vi "111_Auto.vi"() -> ()   [LabVIEW 2020]
uses:
  Global_Variable/Global.vi
  Global_Variable/A131258.vi
panel:
  out "合格":bool=TRUE
  out "Tab Control":enum32{"力特性", "内泄露", "压销位移力曲线"}(tab)
  out "力特性":cluster{dbl[], dbl[]}[](graph)
  out "内泄露":cluster{dbl[], dbl[]}[](graph)
  out "压力位移曲线":cluster{dbl[], dbl[]}[](graph)
  in  "判定结果":bool[][](array[boolean])=[[TRUE]]
  in  "STEP":string
  # "力特性试验"
  # "内泄露试验"
  # "压销位移力曲线"
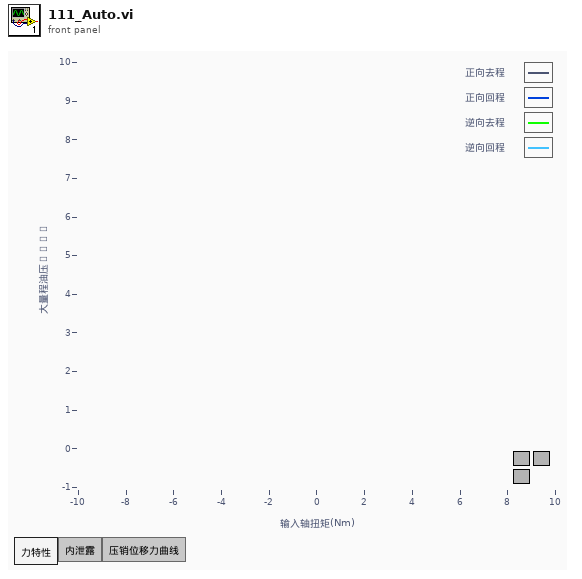
[diagram p1: front panel]
types:
  T1 = typedef "lveventtype.ctl" = enum32{"Null", "Timeout", "Annotation Menu Selection", "Annotation Menu Selection?", "App Instance Close", "App Instance Close?", "Autoscale Range Change", "Bookmark Info Change", "Cell Edit", "Cell Edit?", "Cursor Grab", "Cursor Grab?", "Cursor Menu Selection", "Cursor Menu Selection?", "Cursor Move", "Cursor Release", "Data Change", "Direction Change", "Display State Change", "Drag Ended", "Drag Enter", "Drag Leave", "Drag Over", "Drag Source Update", "Drag Starting", "Drag Starting?", "Drop", "Exec State Change", "Key Down", "Key Down?", "Key Repeat", "Key Repeat?", "Key Up", "Listbox Double Click", "Menu Activation?", "Menu Selection (App)", "Menu Selection? (App)", "Menu Selection (User)", "Mouse Down", "Mouse Down?", "Mouse Enter", "Mouse Leave", "Mouse Move", "Mouse Up", "Mouse Wheel", "NI Security User Change (App)", "Pane Size", "Panel Close", "Panel Close?", "Panel Resize", "Plot Attribute Change", "Scale Range Change", "Shortcut Menu Activation?", "Shortcut Menu Selection (App)", "Shortcut Menu Selection? (App)", "Shortcut Menu Selection (User)", "Tree Double Click", "Tree Drag", "Tree Drag?", "Tree Drop", "Tree Drop?", "Tree Item Close", "Tree Item Close?", "Tree Item Open", "Tree Item Open?", "User Event", "Value Change"}
  T2 = typedef "LVPoint32TypeDef.ctl" = cluster{"Horizontal":i32, "Vertical":i32}
  T3 = cluster{"           对称性":cluster{"下限":dbl, "上限":dbl}, "  正向最大油压":cluster{"下限":dbl, "上限":dbl}, "  逆向最大油压":cluster{"下限":dbl, "上限":dbl}, "定点A正向扭矩":cluster{"下限":dbl, "上限":dbl}, "定点A逆向扭矩":cluster{"下限":dbl, "上限":dbl}, "定点B正向扭矩":cluster{"下限":dbl, "上限":dbl}, "定点B逆向扭矩":cluster{"下限":dbl, "上限":dbl}}
  T4 = cluster{"         对称性":cluster{"下限":dbl, "上限":dbl}, "正向最大角度":cluster{"下限":dbl, "上限":dbl}, "逆向最大角度":cluster{"下限":dbl, "上限":dbl}}
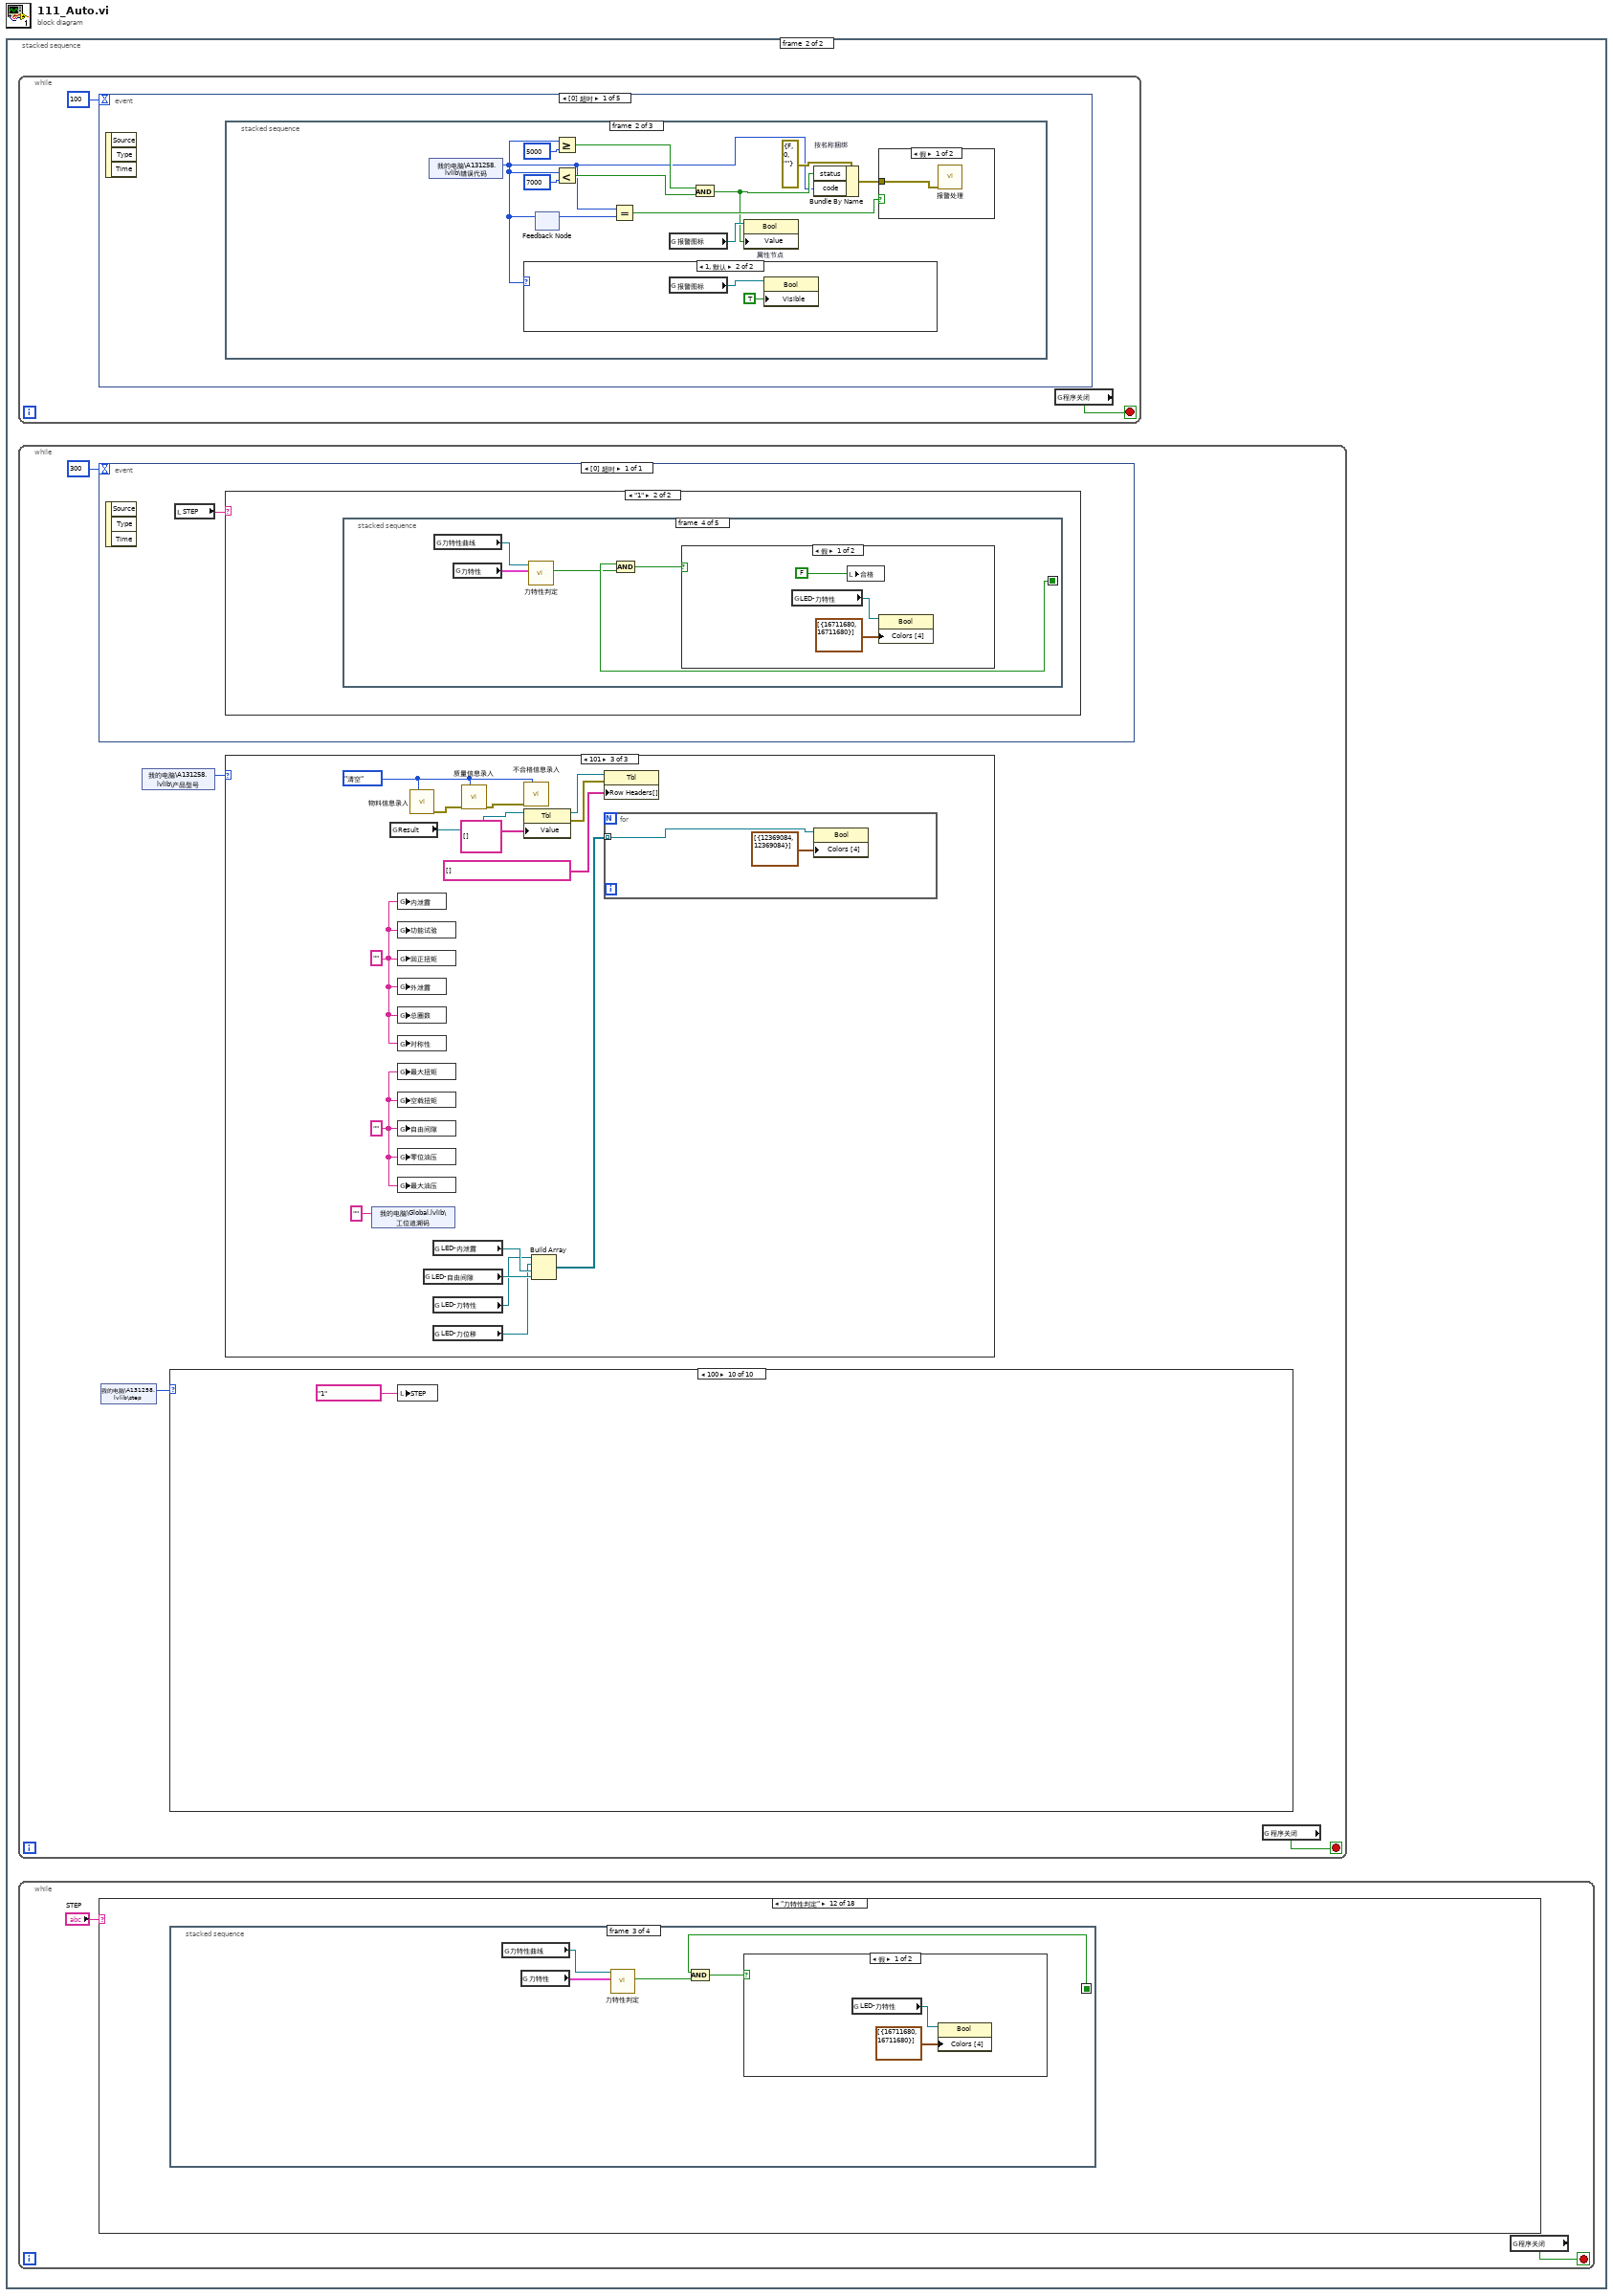
[diagram p0: block diagram]
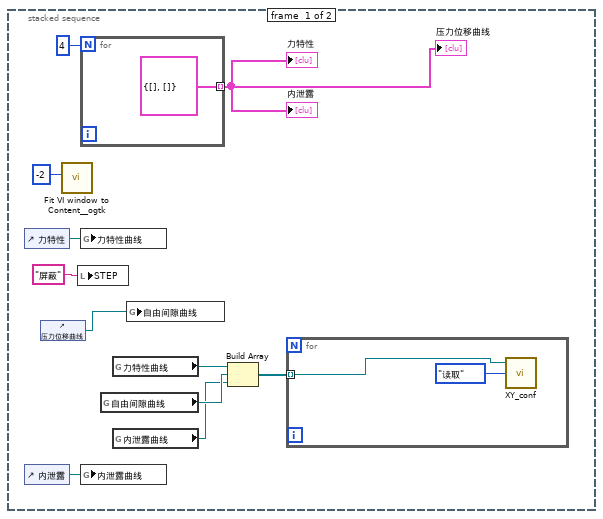
[diagram p2: hidden frame]
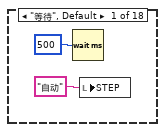
[diagram p3: hidden frame]
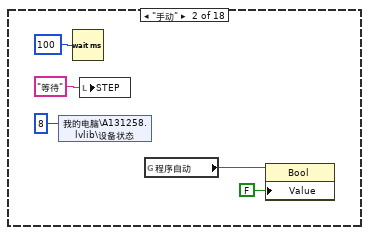
[diagram p4: hidden frame]
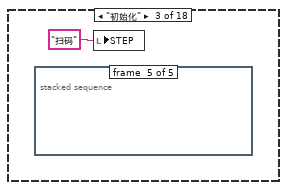
[diagram p5: hidden frame]
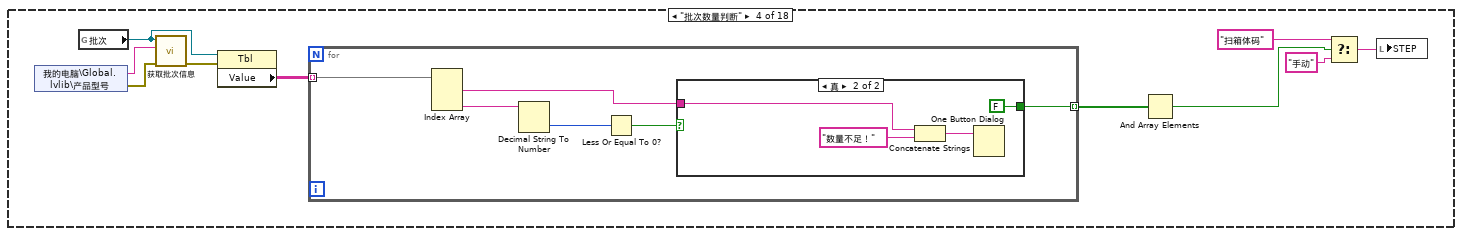
[diagram p10: hidden frame]
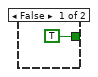
[diagram p11: hidden frame]
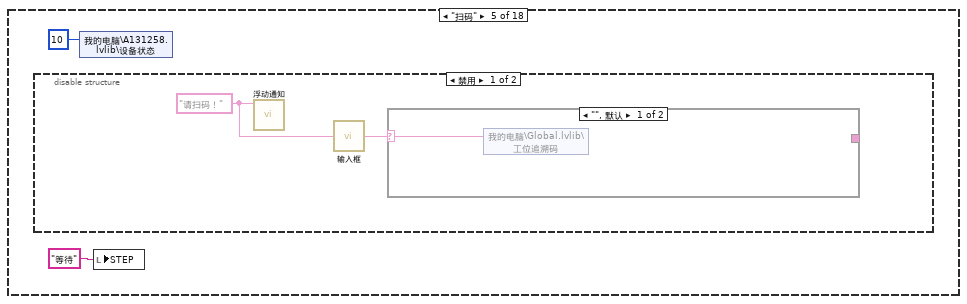
[diagram p12: hidden frame]
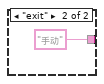
[diagram p13: hidden frame]
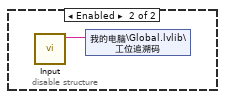
[diagram p14: hidden frame]
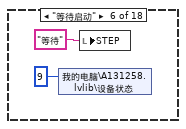
[diagram p15: hidden frame]
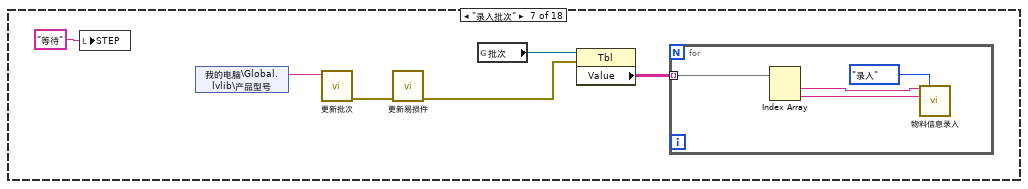
[diagram p16: hidden frame]
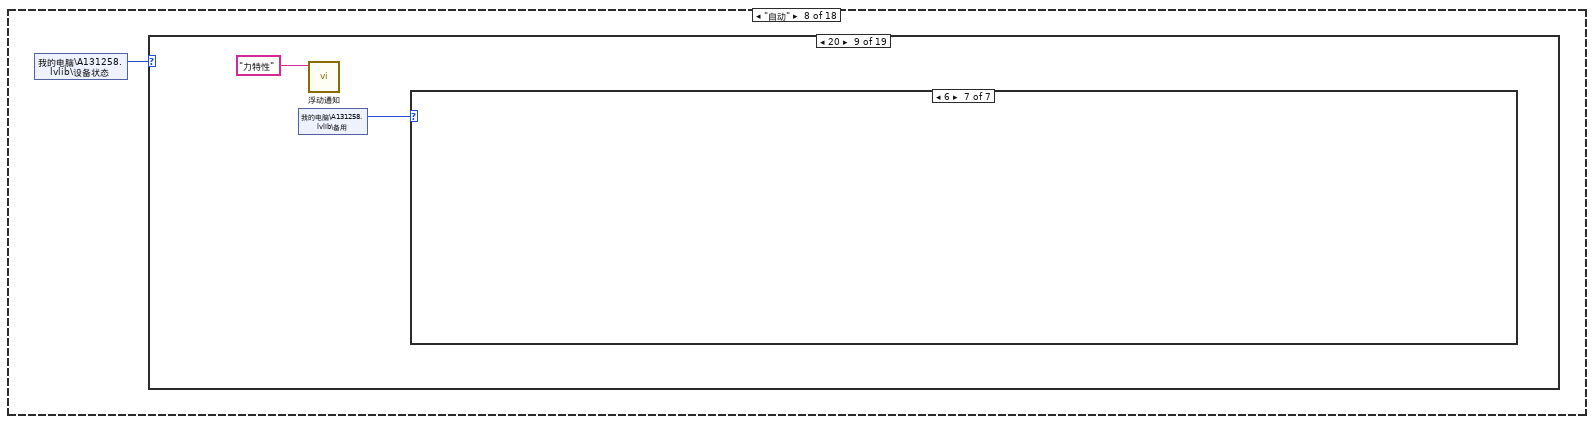
[diagram p17: hidden frame]
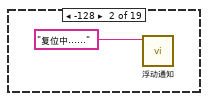
[diagram p19: hidden frame]
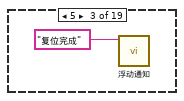
[diagram p20: hidden frame]
diagram:
  n1 = stacked-sequence {
    frame #0 {
      n2 = control-ref of="力特性"() -> (w10:refnum<vi>)
      n3 = control-ref of="内泄露"() -> (w6:refnum<vi>)
      n4 = control-ref of="压力位移曲线"() -> (w9:refnum<vi>)
      n5 = call <userlib>:"Fit VI window to Content__ogtk.vi"("border spacing (2 px)"=-2) -> ()  [unwired: 5 in, 2 out]
      n6 = local write "STEP"("屏蔽" ("STEP")) -> ()
      n7 = for {
        N: 4 -> [_]
        tunnel: [cluster{dbl[], dbl[]} {[], []}] -> w2 mode=indexing
      }
      "压力位移曲线" <- w2
      "力特性" <- w2
      "内泄露" <- w2
      n8 = global write "A131258.vi" "力特性曲线"(w10) -> ()
      n9 = global write "A131258.vi" "内泄露曲线"(w6) -> ()
      n10 = global read "A131258.vi" "自由间隙曲线"() -> (w5:refnum<vi>)
      n11 = global read "A131258.vi" "力特性曲线"() -> (w8:refnum<vi>)
      n12 = global read "A131258.vi" "内泄露曲线"() -> (w4:refnum<vi>)
      n13 = global write "A131258.vi" "自由间隙曲线"(w9) -> ()
      n14 = Build Array(w8, w5, w4) -> (w7:refnum<vi>[])
      n15 = for {
        tunnel: w7 -> [w13] mode=indexing
        n16 = call "XY_conf.vi"("方式"=enum16{"写入", "读取"}."读取", "XY图引用"=w13) -> ()  [unwired: 3 in, 1 out]
      }
    }
    frame #1 {
      n17 = while {
        stop <- w307 stop-if-true
        n18 = event shown="[0] 超时" {
          selector: _ -> [_ _ _ _ _]
          dyn-events: _ -> [_ _ _ _ _]
          timeout: 100 -> [_ _ _ _ _]
          event Timeout {
            n19 = event-data() -> ()  [unwired: 1 in, 3 out]
            n20 = stacked-sequence {
              frame #0 {
                n21 = global read "A131258.vi" "试验项"() -> (→"Tab Control":enum32{"力特性", "内泄露", "压销位移力曲线"})
              }
              frame #1 {
                n22 = shared-variable "我的电脑\\A131258.lvlib\\错误代码"() -> (w310:i16)  [unwired: 1 in, 1 out]
                n23 = case shown="1, 默认" w310 {
                  frame 0 {
                    n24 = global read "Global.vi" "报警图标"() -> (w321:refnum<vi>)
                    n25 = property class="Bool"(reference=w321, "Visible"=FALSE ("可见")) -> ()  [unwired: 1 in, 2 out]
                  }
                  frame 1, Default {
                    n26 = global read "Global.vi" "报警图标"() -> (w324:refnum<vi>)
                    n27 = property class="Bool"(reference=w324, "Visible"=TRUE ("可见")) -> ()  [unwired: 1 in, 2 out]
                  }
                }
                n28 = feedback #1() -> (w320:i16)  [unwired: 1 in]
                n29 = feedback-in #1(w310) -> ()
                n30 = Greater Or Equal?(x=w310, y=i16 5000) -> (x >= y?=w318:bool)
                n31 = Less?(x=w310, y=i16 7000) -> (x < y?=w319:bool)
                n32 = Equal?(x=w310, y=w320) -> (x = y?=w317:bool)
                n33 = global read "Global.vi" "报警图标"() -> (w312:refnum<vi>)
                n34 = And(x=w318, y=w319) -> (x .and. y?=w311:bool)
                n35 = property on="属性节点" class="Bool"(reference=w312, "Value"=w311) -> ()  [unwired: 1 in, 2 out]
                n36 = Bundle By Name "按名称捆绑"(cluster=errorcluster {"status"=FALSE, "code"=0, "source"=""} ("错误常量"), "status"=w311, "code"=w310) -> (w316:errorcluster)
                n37 = case shown="假" w317 {
                  tunnel: w316 -> [w325 _]
                  frame False {
                    n38 = call "报警处理.vi"("错误常量"=w325) -> ()  [unwired: 9 in, 2 out]
                  }
                  frame True {
                  }
                }
              }
              frame #2 {
                n39 = shared-variable "我的电脑\\A131258.lvlib\\自动手动切换"() -> (w326:u16)  [unwired: 1 in, 1 out]
                n40 = case shown="1" w326 {
                  frame 0, Default {
                  }
                  frame 1 {
                    n41 = shared-variable "我的电脑\\A131258.lvlib\\设备状态"() -> (w327:i16)  [unwired: 1 in, 1 out]
                    n42 = case shown="5" w327 {
                      frame Default {
                      }
                      frame 5 {
                      }
                    }
                  }
                }
              }
            }
          }
          event "压力位移曲线", "力特性": Scale Range Change {
            n43 = event-data() -> ("CtlRef"=w328:refnum<vi>)  [unwired: 1 in]
            n44 = call "XY_conf.vi"("方式"=enum16{"写入", "读取"}."写入", "XY图引用"=w328) -> ()  [unwired: 3 in, 1 out]
          }
          event Panel Close {
            n45 = event-data() -> ()  [unwired: 1 in, 4 out]
            n46 = global write "Global.vi" "程序关闭"(TRUE ("程序关闭")) -> ()
          }
          event "压力位移曲线", "力特性": Mouse Enter; "压力位移曲线", "力特性": Mouse Leave; "压力位移曲线", "力特性": Cursor Move {
            n47 = event-data() -> ("CtlRef"=w333:refnum<vi>, "Type"=w331:T1)  [unwired: 1 in]
            n48 = call "CursorShow.vi"("nameShow"=TRUE, "Type"=w331, "Graph"=w333) -> ()  [unwired: 7 in, 2 out]
          }
          event "压力位移曲线", "力特性": Mouse Down {
            n49 = event-data() -> ("CtlRef"=w334:refnum<vi>, "Type"=w337:T1, "Coords"=w336:T2)  [unwired: 1 in]
            n50 = invoke class="XYGraph (严格)" method="Map Coords To XY"(reference=w334, "Coords"=w336) -> ("XY"=w335:cluster{"X":dbl, "Y":dbl})  [unwired: 5 in, 6 out]
            n51 = call "CursorShow.vi"("游标.游标位置"=w335, "Type"=w337, "Graph"=w334) -> ()  [unwired: 7 in, 2 out]
          }
        }
        n52 = global read "Global.vi" "程序关闭"() -> (w307:bool)
      }
      n53 = while {
        stop <- w341 stop-if-true
        n54 = event shown="[0] 超时" {
          selector: _ -> [_]
          dyn-events: _ -> [_]
          timeout: 300 -> [_]
          event Timeout {
            n55 = event-data() -> ()  [unwired: 1 in, 3 out]
            n56 = local read "STEP"() -> (w342:string)
            n57 = case shown="\"1\"" w342 {
              frame "假", Default {
              }
              frame "1" {
                n58 = stacked-sequence {
                  seq-local: [_ _ w358 _ _] -> [_ _ _ w367 _]
                  frame #0 {
                    n59 = local write "STEP"("0" ("STEP")) -> ()
                    n60 = shared-variable "我的电脑\\A131258.lvlib\\step"(i16 101 ("step")) -> ()  [unwired: 1 in, 1 out]
                  }
                  frame #1 {
                    n61 = global read "Global.vi" "Result"() -> (w347:refnum<vi>)
                    n62 = property class="Tbl"(reference=w347) -> (reference out=w350:refnum<vi>, error out=w355:errorcluster, "Row Headers[]"=w348:string[])  [unwired: 1 in]
                    n63 = Build Array (concatenate)(w348, string[] ["力特性"] ("数组")) -> (w349:string[])
                    n64 = property class="Tbl"(reference=w350, error in=w355, "Row Headers[]"=w349) -> (reference out=w351:refnum<vi>, error out=w356:errorcluster)
                    n65 = property class="Tbl"(reference=w351, error in=w356) -> (reference out=w352:refnum<vi>, error out=w357:errorcluster, "Value"=w353:string[][])
                    n66 = Build Array (concatenate)(w353, string[][] [[" "]] ("数组")) -> (w354:string[][])
                    n67 = property class="Tbl"(reference=w352, error in=w357, "Value"=w354) -> ()  [unwired: 2 out]
                  }
                  frame #2 {
                    n68 = shared-variable "我的电脑\\A131258.lvlib\\产品参数"() -> (w362:sgl[])  [unwired: 1 in, 1 out]
                    n69 = global read "A131258.vi" "压力损失"() -> (w359:cluster{"下限":dbl, "上限":dbl})
                    n70 = Index Array(array=w362, index=4 ("索引")) -> (element=w360:sgl)
                    n71 = call "压力损失.vi"("压力损失"=w360, "压力损失判定条件"=w359) -> ("OK"=w358:bool)  [unwired: 7 in, 1 out]
                  }
                  frame #3 {
                    n72 = global read "A131258.vi" "力特性曲线"() -> (w364:refnum<vi>)
                    n73 = global read "A131258.vi" "力特性"() -> (w363:T3)
                    n74 = call "力特性判定.vi"("曲线引用"=w364, "力特性判定条件"=w363) -> ("OK？"=w365:bool)  [unwired: 6 in, 2 out]
                    n75 = And(x=w367, y=w365) -> (x .and. y?=w366:bool)
                    n76 = case shown="假" w366 {
                      frame False {
                        n77 = global read "A131258.vi" "LED-力特性"() -> (w369:refnum<vi>)
                        n78 = local write "合格"(FALSE ("合格")) -> ()
                        n79 = property class="Bool"(reference=w369, "Colors [4]"=cluster{u32, u32}[] [{16711680, 16711680}] ("颜色[4]")) -> ()  [unwired: 1 in, 2 out]
                      }
                      frame True {
                        n80 = global read "A131258.vi" "LED-力特性"() -> (w371:refnum<vi>)
                        n81 = property class="Bool"(reference=w371, "Colors [4]"=cluster{u32, u32}[] [{6618880, 6618880}] ("颜色[4]")) -> ()  [unwired: 1 in, 2 out]
                      }
                    }
                  }
                  frame #4 {
                  }
                }
              }
            }
          }
        }
        n82 = shared-variable "我的电脑\\A131258.lvlib\\step"() -> (w340:i16)  [unwired: 1 in, 1 out]
        n83 = shared-variable "我的电脑\\A131258.lvlib\\产品型号"() -> (w339:i16)  [unwired: 1 in, 1 out]
        n84 = case shown="100" w340 {
          frame 0, Default {
          }
          frame 1 {
            n85 = call "浮动通知.vi"("通知内容"="复位完成" ("Status")) -> ()  [unwired: 11 in]
          }
          frame 2 {
            n86 = call "浮动通知.vi"("通知内容"="请启动！" ("Status")) -> ()  [unwired: 11 in]
          }
          frame 3 {
            n87 = call "浮动通知.vi"("通知内容"="手动状态！" ("Status")) -> ()  [unwired: 11 in]
          }
          frame 4 {
            n88 = global read "Global.vi" "试验项目"() -> (w399:bool[])
            n89 = local read "压力位移曲线"() -> (w398:cluster{dbl[], dbl[]}[])
            n90 = call "浮动通知.vi"("通知内容"="力位移曲线" ("Status")) -> ()  [unwired: 11 in]
            n91 = for {
              tunnel: w399 -> [w417] mode=indexing
              i -> [w418]
              n92 = case shown="0" w418 {
                tunnel: w417 -> [_ w419]
                frame Default {
                }
                frame 0 {
                  n93 = case shown="真" w419 {
                    frame False {
                    }
                    frame True {
                      n94 = global write "A131258.vi" "试验项"(enum32{"力特性", "内泄露", "压销位移力曲线"}."压销位移力曲线" ("试验项")) -> ()
                    }
                  }
                }
              }
            }
            n95 = for {
              tunnel: [w403] -> w397 mode=indexing
              tunnel: w398 -> [w402] mode=indexing
              i -> [w401]
              n96 = case shown="0" w401 {
                tunnel: [w404 w408] -> w403
                tunnel: w402 -> [w404 w407]
                frame Default {
                }
                frame 0 {
                  n97 = Unbundle(w407) -> (w412:dbl[], w411:dbl[])
                  n98 = shared-variable "我的电脑\\A131258.lvlib\\压销力"() -> (w416:sgl[])  [unwired: 1 in, 1 out]
                  n99 = shared-variable "我的电脑\\A131258.lvlib\\压销位移"() -> (w414:sgl[])  [unwired: 1 in, 1 out]
                  n100 = Index Array(array=w416, index=4) -> (element=w406:sgl)
                  n101 = Build Array (concatenate)(w411, w406) -> (w409:dbl[])
                  n102 = Index Array(array=w414, index=4) -> (element=w405:sgl)
                  n103 = Build Array (concatenate)(w412, w405) -> (w410:dbl[])
                  n104 = Bundle(w410, w409) -> (w408:cluster{dbl[], dbl[]})  [unwired: 1 in]
                }
              }
            }
            n105 = local write "压力位移曲线"(w397) -> ()
          }
          frame 5 {
            n106 = global read "Global.vi" "试验项目"() -> (w421:bool[])
            n107 = local read "力特性"() -> (w423:cluster{dbl[], dbl[]}[])
            n108 = call "浮动通知.vi"("通知内容"="力特性" ("Status")) -> ()  [unwired: 11 in]
            n109 = for {
              tunnel: w421 -> [w425] mode=indexing
              i -> [w426]
              n110 = case shown="0" w426 {
                tunnel: w425 -> [_ w427]
                frame Default {
                }
                frame 0 {
                  n111 = case shown="真" w427 {
                    frame False {
                    }
                    frame True {
                      n112 = global write "A131258.vi" "试验项"(enum32{"力特性", "内泄露", "压销位移力曲线"}."力特性" ("试验项")) -> ()
                    }
                  }
                }
              }
            }
            n113 = for {
              tunnel: [w431] -> w422 mode=indexing
              tunnel: w423 -> [w430] mode=indexing
              i -> [w429]
              n114 = case shown="0" w429 {
                tunnel: [w432 w436] -> w431
                tunnel: w430 -> [w432 w435]
                frame Default {
                }
                frame 0 {
                  n115 = Unbundle(w435) -> (w440:dbl[], w439:dbl[])
                  n116 = shared-variable "我的电脑\\A131258.lvlib\\油压传感器(大量程)"() -> (w444:sgl[])  [unwired: 1 in, 1 out]
                  n117 = shared-variable "我的电脑\\A131258.lvlib\\输入轴扭矩传感器"() -> (w442:sgl[])  [unwired: 1 in, 1 out]
                  n118 = Index Array(array=w442, index=4) -> (element=w433:sgl)
                  n119 = Index Array(array=w444, index=4) -> (element=w434:sgl)
                  n120 = Build Array (concatenate)(w440, w433) -> (w438:dbl[])
                  n121 = Build Array (concatenate)(w439, w434) -> (w437:dbl[])
                  n122 = Bundle(w438, w437) -> (w436:cluster{dbl[], dbl[]})  [unwired: 1 in]
                }
              }
            }
            n123 = local write "力特性"(w422) -> ()
          }
          frame 6 {
            n124 = global read "Global.vi" "试验项目"() -> (w448:bool[])
            n125 = local read "内泄露"() -> (w447:cluster{dbl[], dbl[]}[])
            n126 = call "浮动通知.vi"("通知内容"="内泄露" ("Status")) -> ()  [unwired: 11 in]
            n127 = for {
              tunnel: w448 -> [w465] mode=indexing
              i -> [w466]
              n128 = case shown="0" w466 {
                tunnel: w465 -> [_ w467]
                frame Default {
                }
                frame 0 {
                  n129 = case shown="真" w467 {
                    frame False {
                    }
                    frame True {
                      n130 = global write "A131258.vi" "试验项"(enum32{"力特性", "内泄露", "压销位移力曲线"}."内泄露" ("试验项")) -> ()
                    }
                  }
                }
              }
            }
            n131 = for {
              tunnel: [w451] -> w446 mode=indexing
              tunnel: w447 -> [w450] mode=indexing
              i -> [w449]
              n132 = case shown="0" w449 {
                tunnel: [w452 w458] -> w451
                tunnel: w450 -> [w452 w457]
                frame Default {
                }
                frame 0 {
                  n133 = Unbundle(w457) -> (w462:dbl[], w461:dbl[])
                  n134 = shared-variable "我的电脑\\A131258.lvlib\\内泄露参数"() -> (w464:sgl[])  [unwired: 1 in, 1 out]
                  n135 = shared-variable "我的电脑\\A131258.lvlib\\内泄露保持时间1"() -> (w453:sgl)  [unwired: 1 in, 1 out]
                  n136 = Index Array(array=w464, index=4) -> (element=w456:sgl)
                  n137 = Build Array (concatenate)(w461, w456) -> (w459:dbl[])
                  n138 = Divide(x=w453, y=sgl 1000.0) -> (x/y=w455:sgl)
                  n139 = Build Array (concatenate)(w462, w455) -> (w460:dbl[])
                  n140 = Bundle(w460, w459) -> (w458:cluster{dbl[], dbl[]})  [unwired: 1 in]
                }
              }
            }
            n141 = local write "内泄露"(w446) -> ()
          }
          frame 7 {
            n142 = global read "Global.vi" "试验项目"() -> (w472:bool[])
            n143 = local read "内泄露"() -> (w470:cluster{dbl[], dbl[]}[])
            n144 = call "浮动通知.vi"("通知内容"="内泄露" ("Status")) -> ()  [unwired: 11 in]
            n145 = for {
              tunnel: w472 -> [w489] mode=indexing
              i -> [w490]
              n146 = case shown="0" w490 {
                tunnel: w489 -> [_ w491]
                frame Default {
                }
                frame 0 {
                  n147 = case shown="真" w491 {
                    frame False {
                    }
                    frame True {
                      n148 = global write "A131258.vi" "试验项"(enum32{"力特性", "内泄露", "压销位移力曲线"}."内泄露" ("试验项")) -> ()
                    }
                  }
                }
              }
            }
            n149 = for {
              tunnel: [w475] -> w469 mode=indexing
              tunnel: w470 -> [w474] mode=indexing
              i -> [w473]
              n150 = case shown="默认" w473 {
                tunnel: [w476 w482] -> w475
                tunnel: w474 -> [w476 w481]
                frame Default {
                }
                frame 1 {
                  n151 = Unbundle(w481) -> (w486:dbl[], w485:dbl[])
                  n152 = shared-variable "我的电脑\\A131258.lvlib\\内泄露参数"() -> (w488:sgl[])  [unwired: 1 in, 1 out]
                  n153 = shared-variable "我的电脑\\A131258.lvlib\\内泄露保持时间1"() -> (w477:sgl)  [unwired: 1 in, 1 out]
                  n154 = Index Array(array=w488, index=4) -> (element=w480:sgl)
                  n155 = Build Array (concatenate)(w485, w480) -> (w483:dbl[])
                  n156 = Divide(x=w477, y=u32 1000) -> (x/y=w478:sgl)
                  n157 = Build Array (concatenate)(w486, w478) -> (w484:dbl[])
                  n158 = Bundle(w484, w483) -> (w482:cluster{dbl[], dbl[]})  [unwired: 1 in]
                }
              }
            }
            n159 = local write "内泄露"(w469) -> ()
          }
          frame 15 {
            n160 = call "浮动通知.vi"("通知内容"="报表生成中" ("Status")) -> ()  [unwired: 11 in]
            n161 = call "Report.vi"() -> ()  [unwired: 11 in, 1 out]
          }
          frame 100 {
            n162 = local write "STEP"("1" ("STEP")) -> ()
          }
        }
        n163 = case shown="101" w339 {
          frame 0, Default {
          }
          frame 100 {
            n164 = for {
              N: 4 -> [_]
              tunnel: [cluster{dbl[], dbl[]} {[], []}] -> w374 mode=indexing
            }
            n165 = local write "力特性"(w374) -> ()
            n166 = local write "压力位移曲线"(w374) -> ()
            n167 = local write "内泄露"(w374) -> ()
          }
          frame 101 {
            w378 = enum16{"录入", "清空"}."清空" ("功能")
            w386 = "" ("最大油压")
            w385 = "" ("内泄露")
            n168 = shared-variable "我的电脑\\Global.lvlib\\工位追溯码"("" ("传感器码")) -> ()  [unwired: 1 in, 1 out]
            n169 = global read "Global.vi" "Result"() -> (w384:refnum<vi>)
            n170 = global write "检测结果.vi" "内泄露"(w385) -> ()
            n171 = global write "检测结果.vi" "功能试验"(w385) -> ()
            n172 = global write "检测结果.vi" "回正扭矩"(w385) -> ()
            n173 = global write "检测结果.vi" "外泄露"(w385) -> ()
            n174 = global write "检测结果.vi" "总圈数"(w385) -> ()
            n175 = global write "检测结果.vi" "对称性"(w385) -> ()
            n176 = global write "检测结果.vi" "最大扭矩"(w386) -> ()
            n177 = global write "检测结果.vi" "空载扭矩"(w386) -> ()
            n178 = global write "检测结果.vi" "自由间隙"(w386) -> ()
            n179 = global write "检测结果.vi" "零位油压"(w386) -> ()
            n180 = global write "检测结果.vi" "最大油压"(w386) -> ()
            n181 = call "物料信息录入.vi"("功能"=w378) -> ("错误输出"=w381:errorcluster)  [unwired: 14 in]
            n182 = global read "A131258.vi" "LED-自由间隙"() -> (w390:refnum<vi>)
            n183 = global read "A131258.vi" "LED-内泄露"() -> (w389:refnum<vi>)
            n184 = global read "A131258.vi" "LED-力特性"() -> (w387:refnum<vi>)
            n185 = global read "A131258.vi" "LED-力位移"() -> (w388:refnum<vi>)
            n186 = call "质量信息录入.vi"("功能"=w378, "错误输入（无错误）"=w381) -> ("错误输出"=w380:errorcluster)  [unwired: 13 in]
            n187 = call "不合格信息录入.vi"("功能"=w378, "错误输入（无错误）"=w380) -> ()  [unwired: 13 in, 1 out]
            n188 = property class="Tbl"(reference=w384, "Value"=string[][] []) -> (reference out=w383:refnum<vi>, error out=w382:errorcluster)  [unwired: 1 in]
            n189 = Build Array(w387, w388, w389, w390) -> (w391:refnum<vi>[])
            n190 = property class="Tbl"(reference=w383, error in=w382, "Row Headers[]"=string[] [] ("列首字符串[]")) -> ()  [unwired: 2 out]
            n191 = for {
              tunnel: w391 -> [w392] mode=indexing
              n192 = property class="Bool"(reference=w392, "Colors [4]"=cluster{u32, u32}[] [{12369084, 12369084}] ("颜色[4]")) -> ()  [unwired: 1 in, 2 out]
            }
          }
        }
        n193 = global read "Global.vi" "程序关闭"() -> (w341:bool)
      }
      n194 = while {
        stop <- w15 stop-if-true
        n195 = case shown="\"力特性判定\"" "STEP" {
          frame "等待", Default {
            n196 = Wait (ms)(milliseconds to wait=u32 500 ("等待时间（毫秒）")) -> ()  [unwired: 1 out]
            n197 = local write "STEP"("自动" ("STEP")) -> ()
          }
          frame "手动" {
            n198 = shared-variable "我的电脑\\A131258.lvlib\\设备状态"(u16 8 ("设备状态")) -> ()  [unwired: 1 in, 1 out]
            n199 = Wait (ms)(milliseconds to wait=u32 100 ("等待时间（毫秒）")) -> ()  [unwired: 1 out]
            n200 = local write "STEP"("等待" ("STEP")) -> ()
            n201 = global read "Global.vi" "程序自动"() -> (w21:refnum<vi>)
            n202 = property class="Bool"(reference=w21, "Value"=FALSE) -> ()  [unwired: 1 in, 2 out]
          }
          frame "初始化" {
            n203 = stacked-sequence {
              frame #0 {
              }
              frame #1 {
              }
              frame #2 {
              }
              frame #3 {
              }
              frame #4 {
              }
            }
            n204 = local write "STEP"("扫码" ("STEP")) -> ()
          }
          frame "批次数量判断" {
            n205 = shared-variable "我的电脑\\Global.lvlib\\产品型号"() -> (w30:string, error out=w33:errorcluster)  [unwired: 1 in]
            n206 = global read "Global.vi" "批次"() -> (w31:refnum<vi>)
            n207 = call "获取批次信息.vi"("error in (no error)"=w33, "产品型号"=w30, "Tbl引用句柄"=w31) -> ("error out"=w32:errorcluster)  [unwired: 7 in, 1 out]
            n208 = property class="Tbl"(reference=w31, error in=w32) -> ("Value"=w34:string[][])  [unwired: 2 out]
            n209 = for {
              tunnel: w34 -> [w40] mode=indexing
              tunnel: [w35] -> w29 mode=indexing
              n210 = Index Array(array=w40) -> (element #1=w36:string, element #3=w39:string)  [unwired: 3 in, 1 out]
              n211 = Decimal String To Number(string=w39) -> (number=w38:i32)  [unwired: 2 in, 1 out]
              n212 = Less Or Equal To 0?(x=w38) -> (x <= 0?=w37:bool)
              n213 = case shown="真" w37 {
                tunnel: w36 -> [_ w45]
                tunnel: [TRUE FALSE] -> w35
                frame False {
                }
                frame True {
                  n214 = Concatenate Strings(w45, "数量不足！" ("字符串")) -> (w43:string)
                  n215 = One Button Dialog(message=w43) -> ()  [unwired: 1 in, 1 out]
                }
              }
            }
            n216 = And Array Elements(Boolean array=w29) -> (logical AND=w28:bool)
            n217 = Select(t="扫箱体码" ("STEP"), s=w28, f="手动" ("STEP")) -> (s? t:f=w25:string)
            n218 = local write "STEP"(w25) -> ()
          }
          frame "扫码" {
            n219 = disable-structure shown="禁用" {
              frame Disabled {
                w48 = "请扫码！" ("提示信息")
                n220 = call "浮动通知.vi"("通知内容"=w48) -> ()  [unwired: 11 in]
                n221 = call "输入框.vi"("提示信息"=w48) -> ("条形码输出"=w49:string)
                n222 = case shown="\"\", 默认" w49 {
                  selector: w49 -> [w50 _]
                  tunnel: [_ "手动"] -> _
                  frame "", Default {
                    n223 = shared-variable "我的电脑\\Global.lvlib\\工位追溯码"(w50) -> ()  [unwired: 1 in, 1 out]
                  }
                  frame "exit" {
                  }
                }
              }
              frame Enabled {
                n224 = call "Input.vi"() -> ("产品编号"=w52:string)  [unwired: 11 in]
                n225 = shared-variable "我的电脑\\Global.lvlib\\工位追溯码"(w52) -> ()  [unwired: 1 in, 1 out]
              }
            }
            n226 = shared-variable "我的电脑\\A131258.lvlib\\设备状态"(i16 10 ("设备状态")) -> ()  [unwired: 1 in, 1 out]
            n227 = local write "STEP"("等待" ("State(s) in Front (\"\")")) -> ()
          }
          frame "等待启动" {
            n228 = shared-variable "我的电脑\\A131258.lvlib\\设备状态"(i16 9 ("设备状态控制字")) -> ()  [unwired: 1 in, 1 out]
            n229 = local write "STEP"("等待" ("State(s) in Front (\"\")")) -> ()
          }
          frame "录入批次" {
            n230 = local write "STEP"("等待" ("STEP")) -> ()
            n231 = shared-variable "我的电脑\\Global.lvlib\\产品型号"() -> (w56:string)  [unwired: 1 in, 1 out]
            n232 = call "更新批次.vi"("型号"=w56) -> ("error out"=w57:errorcluster)  [unwired: 10 in]
            n233 = call "更新易损件.vi"("error in (no error)"=w57) -> ("error out"=w60:errorcluster)  [unwired: 10 in]
            n234 = global read "Global.vi" "批次"() -> (w58:refnum<vi>)
            n235 = property class="Tbl"(reference=w58, error in=w60) -> ("Value"=w59:string[][])  [unwired: 2 out]
            n236 = for {
              tunnel: w59 -> [w63] mode=indexing
              n237 = Index Array(array=w63) -> (element #1=w62:string, element #2=w61:string)  [unwired: 2 in]
              n238 = call "物料信息录入.vi"("物料名称"=w62, "功能"=enum16{"录入", "清空"}."录入", "物料编码"=w61) -> ()  [unwired: 12 in, 1 out]
            }
          }
          frame "自动" {
            n239 = shared-variable "我的电脑\\A131258.lvlib\\设备状态"() -> (w65:i16)  [unwired: 1 in, 1 out]
            n240 = case shown="20" w65 {
              frame Default {
              }
              frame -128 {
                n241 = call "浮动通知.vi"("通知内容"="复位中……" ("Status")) -> ()  [unwired: 11 in]
              }
              frame 5 {
                n242 = call "浮动通知.vi"("通知内容"="复位完成" ("Status")) -> ()  [unwired: 11 in]
              }
              frame 8 {
                n243 = call "浮动通知.vi"("通知内容"="程序停止！" ("Status")) -> ()  [unwired: 11 in]
              }
              frame 0 {
              }
              frame 9 {
                n244 = call "浮动通知.vi"("通知内容"="请启动！" ("Status")) -> ()  [unwired: 11 in]
              }
              frame 10 {
                n245 = call "浮动通知.vi"("通知内容"="套花键" ("Status")) -> ()  [unwired: 11 in]
              }
              frame 11 {
                n246 = local write "STEP"("试验项-力特性" ("STEP")) -> ()
              }
              frame 20 {
                n247 = shared-variable "我的电脑\\A131258.lvlib\\备用"() -> (w72:i16)  [unwired: 1 in, 1 out]
                n248 = call "浮动通知.vi"("通知内容"="力特性" ("Status")) -> ()  [unwired: 11 in]
                n249 = case shown="6" w72 {
                  frame 0, Default {
                  }
                  frame 1 {
                    n250 = local read "力特性"() -> (w74:cluster{dbl[], dbl[]}[])
                    n251 = for {
                      tunnel: [w78] -> w75 mode=indexing
                      tunnel: w74 -> [w77] mode=indexing
                      i -> [w76]
                      n252 = case shown="0" w76 {
                        tunnel: [w79 w83] -> w78
                        tunnel: w77 -> [w79 w82]
                        frame Default {
                        }
                        frame 0 {
                          n253 = Unbundle(w82) -> (w87:dbl[], w86:dbl[])
                          n254 = shared-variable "我的电脑\\A131258.lvlib\\油压传感器(大量程)"() -> (w91:sgl[])  [unwired: 1 in, 1 out]
                          n255 = shared-variable "我的电脑\\A131258.lvlib\\输入轴扭矩传感器"() -> (w89:sgl[])  [unwired: 1 in, 1 out]
                          n256 = Index Array(array=w91, index=4) -> (element=w81:sgl)
                          n257 = Index Array(array=w89, index=4) -> (element=w80:sgl)
                          n258 = Build Array (concatenate)(w87, w80) -> (w85:dbl[])
                          n259 = Build Array (concatenate)(w86, w81) -> (w84:dbl[])
                          n260 = Bundle(w85, w84) -> (w83:cluster{dbl[], dbl[]})  [unwired: 1 in]
                        }
                      }
                    }
                    n261 = local write "力特性"(w75) -> ()
                  }
                  frame 2 {
                    n262 = local read "力特性"() -> (w92:cluster{dbl[], dbl[]}[])
                    n263 = for {
                      tunnel: [w96] -> w93 mode=indexing
                      tunnel: w92 -> [w95] mode=indexing
                      i -> [w94]
                      n264 = case shown="1" w94 {
                        tunnel: [w97 w101] -> w96
                        tunnel: w95 -> [w97 w100]
                        frame Default {
                        }
                        frame 1 {
                          n265 = Unbundle(w100) -> (w105:dbl[], w104:dbl[])
                          n266 = shared-variable "我的电脑\\A131258.lvlib\\油压传感器(大量程)"() -> (w109:sgl[])  [unwired: 1 in, 1 out]
                          n267 = shared-variable "我的电脑\\A131258.lvlib\\输入轴扭矩传感器"() -> (w107:sgl[])  [unwired: 1 in, 1 out]
                          n268 = Index Array(array=w109, index=4) -> (element=w99:sgl)
                          n269 = Index Array(array=w107, index=4) -> (element=w98:sgl)
                          n270 = Build Array (concatenate)(w105, w98) -> (w103:dbl[])
                          n271 = Build Array (concatenate)(w104, w99) -> (w102:dbl[])
                          n272 = Bundle(w103, w102) -> (w101:cluster{dbl[], dbl[]})  [unwired: 1 in]
                        }
                      }
                    }
                    n273 = local write "力特性"(w93) -> ()
                  }
                  frame 3 {
                  }
                  frame 4 {
                    n274 = local read "力特性"() -> (w110:cluster{dbl[], dbl[]}[])
                    n275 = for {
                      tunnel: [w114] -> w111 mode=indexing
                      tunnel: w110 -> [w113] mode=indexing
                      i -> [w112]
                      n276 = case shown="3" w112 {
                        tunnel: [w115 w119] -> w114
                        tunnel: w113 -> [w115 w118]
                        frame Default {
                        }
                        frame 3 {
                          n277 = Unbundle(w118) -> (w123:dbl[], w122:dbl[])
                          n278 = shared-variable "我的电脑\\A131258.lvlib\\油压传感器(大量程)"() -> (w127:sgl[])  [unwired: 1 in, 1 out]
                          n279 = shared-variable "我的电脑\\A131258.lvlib\\输入轴扭矩传感器"() -> (w125:sgl[])  [unwired: 1 in, 1 out]
                          n280 = Index Array(array=w127, index=4) -> (element=w117:sgl)
                          n281 = Index Array(array=w125, index=4) -> (element=w116:sgl)
                          n282 = Build Array (concatenate)(w123, w116) -> (w121:dbl[])
                          n283 = Build Array (concatenate)(w122, w117) -> (w120:dbl[])
                          n284 = Bundle(w121, w120) -> (w119:cluster{dbl[], dbl[]})  [unwired: 1 in]
                        }
                      }
                    }
                    n285 = local write "力特性"(w111) -> ()
                  }
                  frame 5 {
                  }
                  frame 6 {
                  }
                }
              }
              frame 21 {
                n286 = local write "STEP"("力特性判定" ("STEP")) -> ()
                n287 = call "浮动通知.vi"("通知内容"="力特性判定" ("Status")) -> ()  [unwired: 11 in]
              }
              frame 30 {
                n288 = shared-variable "我的电脑\\A131258.lvlib\\备用"() -> (w130:i16)  [unwired: 1 in, 1 out]
                n289 = call "浮动通知.vi"("通知内容"="自由间隙" ("Status")) -> ()  [unwired: 11 in]
                n290 = case shown="1" w130 {
                  frame 0, Default {
                  }
                  frame 1 {
                    n291 = local read "压力位移曲线"() -> (w132:cluster{dbl[], dbl[]}[])
                    n292 = for {
                      tunnel: [w136] -> w133 mode=indexing
                      tunnel: w132 -> [w135] mode=indexing
                      i -> [w134]
                      n293 = case shown="0" w134 {
                        tunnel: [w137 w141] -> w136
                        tunnel: w135 -> [w137 w140]
                        frame Default {
                        }
                        frame 0 {
                          n294 = Unbundle(w140) -> (w145:dbl[], w144:dbl[])
                          n295 = shared-variable "我的电脑\\A131258.lvlib\\压销力"() -> (w147:sgl[])  [unwired: 1 in, 1 out]
                          n296 = shared-variable "我的电脑\\A131258.lvlib\\压销位移"() -> (w149:sgl[])  [unwired: 1 in, 1 out]
                          n297 = Index Array(array=w147, index=0) -> (element=w139:sgl)
                          n298 = Build Array (concatenate)(w145, w139) -> (w143:dbl[])
                          n299 = Index Array(array=w149, index=4) -> (element=w138:sgl)
                          n300 = Build Array (concatenate)(w144, w138) -> (w142:dbl[])
                          n301 = Bundle(w143, w142) -> (w141:cluster{dbl[], dbl[]})  [unwired: 1 in]
                        }
                      }
                    }
                    n302 = local write "压力位移曲线"(w133) -> ()
                  }
                }
              }
              frame 31 {
                n303 = local write "STEP"("自由间隙判定" ("STEP")) -> ()
                n304 = call "浮动通知.vi"("通知内容"="自由间隙判定" ("Status")) -> ()  [unwired: 11 in]
              }
              frame 41 {
                n305 = local write "STEP"("合格判定" ("STEP")) -> ()
                n306 = call "浮动通知.vi"("通知内容"="检测完成" ("Status")) -> ()  [unwired: 11 in]
              }
              frame 100 {
                n307 = global read "Global.vi" "生产数量"() -> (w155:i32)
                n308 = local write "STEP"("初始化" ("STEP")) -> ()
                n309 = Increment(x=w155) -> (x+1=w156:i32)
                n310 = global write "Global.vi" "生产数量"(w156) -> ()
                "合格" <- TRUE ("合格")
              }
              frame 999 {
                n311 = call "浮动通知.vi"("通知内容"="光栅被遮挡，程序暂停，请按复位键继续" ("Status")) -> ()  [unwired: 11 in]
              }
              frame 1024 {
                n312 = call "浮动通知.vi"("通知内容"="急停！" ("Status")) -> ()  [unwired: 11 in]
              }
              frame 3721 {
                n313 = local write "STEP"("不合格锁定" ("STEP")) -> ()
                n314 = call "浮动通知.vi"("通知内容"="产品不合格程序锁定！" ("Status")) -> ()  [unwired: 11 in]
              }
              frame 3722 {
                n315 = global read "Global.vi" "程序自动"() -> (w163:refnum<vi>)
                n316 = property class="Bool"(reference=w163, "Value"=FALSE) -> ()  [unwired: 1 in, 2 out]
                n317 = call "浮动通知.vi"("通知内容"="授权成功，请复位！" ("Status")) -> ()  [unwired: 11 in]
              }
              frame 3723 {
                n318 = call "浮动通知.vi"("通知内容"="请取出不合格产品并摆放至不合格品区！" ("Status")) -> ()  [unwired: 11 in]
              }
            }
          }
          frame "屏蔽" {
          }
          frame "试验项-力特性" {
            n319 = global read "Global.vi" "试验项目"() -> (w166:bool[])
            n320 = for {
              tunnel: w166 -> [w167] mode=indexing
              i -> [w168]
              n321 = case shown="0" w168 {
                tunnel: w167 -> [_ w169]
                frame Default {
                }
                frame 0 {
                  n322 = case shown="假" w169 {
                    frame False {
                      n323 = local write "STEP"("试验项-自由间隙" ("STEP")) -> ()
                    }
                    frame True {
                      n324 = shared-variable "我的电脑\\A131258.lvlib\\设备状态"(i16 20 ("设备状态")) -> ()  [unwired: 1 in, 1 out]
                      n325 = local write "STEP"("等待" ("STEP")) -> ()
                      n326 = global write "A131258.vi" "试验项"(enum32{"力特性", "内泄露", "压销位移力曲线"}."力特性" ("试验项")) -> ()
                    }
                  }
                }
              }
            }
          }
          frame "试验项-自由间隙" {
            n327 = global read "Global.vi" "试验项目"() -> (w174:bool[])
            n328 = for {
              tunnel: w174 -> [w175] mode=indexing
              i -> [w176]
              n329 = case shown="3" w176 {
                tunnel: w175 -> [_ w177]
                frame Default {
                }
                frame 3 {
                  n330 = case shown="真" w177 {
                    frame False {
                      n331 = shared-variable "我的电脑\\A131258.lvlib\\设备状态"(i16 40 ("设备状态")) -> ()  [unwired: 1 in, 1 out]
                      n332 = local write "STEP"("等待" ("STEP")) -> ()
                    }
                    frame True {
                      n333 = shared-variable "我的电脑\\A131258.lvlib\\设备状态"(i16 30 ("设备状态")) -> ()  [unwired: 1 in, 1 out]
                      n334 = local write "STEP"("等待" ("STEP")) -> ()
                      n335 = global write "A131258.vi" "试验项"(enum32{"力特性", "内泄露", "压销位移力曲线"}."压销位移力曲线" ("试验项")) -> ()
                    }
                  }
                }
              }
            }
          }
          frame "力特性判定" {
            n336 = stacked-sequence {
              seq-local: [_ w196 _ _] -> [_ _ w205 _]
              frame #0 {
                n337 = global read "Global.vi" "Result"() -> (w183:refnum<vi>)
                n338 = property class="Tbl"(reference=w183) -> (reference out=w186:refnum<vi>, error out=w193:errorcluster, "Row Headers[]"=w184:string[])  [unwired: 1 in]
                n339 = Build Array (concatenate)(w184, string[] ["力特性"] ("数组")) -> (w185:string[])
                n340 = property class="Tbl"(reference=w186, error in=w193, "Row Headers[]"=w185) -> (reference out=w187:refnum<vi>, error out=w194:errorcluster)
                n341 = property class="Tbl"(reference=w187, error in=w194) -> (reference out=w189:refnum<vi>, error out=w195:errorcluster, "Value"=w190:string[][])
                n342 = Build Array (concatenate)(w190, string[][] [[" "]] ("数组")) -> (w191:string[][])
                n343 = property class="Tbl"(reference=w189, error in=w195, "Value"=w191) -> ()  [unwired: 2 out]
              }
              frame #1 {
                n344 = shared-variable "我的电脑\\A131258.lvlib\\产品参数"() -> (w200:sgl[])  [unwired: 1 in, 1 out]
                n345 = global read "A131258.vi" "压力损失"() -> (w197:cluster{"下限":dbl, "上限":dbl})
                n346 = Index Array(array=w200, index=4 ("索引")) -> (element=w198:sgl)
                n347 = call "压力损失.vi"("压力损失"=w198, "压力损失判定条件"=w197) -> ("OK"=w196:bool)  [unwired: 7 in, 1 out]
              }
              frame #2 {
                n348 = global read "A131258.vi" "力特性曲线"() -> (w202:refnum<vi>)
                n349 = global read "A131258.vi" "力特性"() -> (w201:T3)
                n350 = call "力特性判定.vi"("曲线引用"=w202, "力特性判定条件"=w201) -> ("OK？"=w203:bool)  [unwired: 6 in, 2 out]
                n351 = And(x=w205, y=w203) -> (x .and. y?=w204:bool)
                n352 = case shown="假" w204 {
                  frame False {
                    n353 = global read "A131258.vi" "LED-力特性"() -> (w206:refnum<vi>)
                    n354 = property class="Bool"(reference=w206, "Colors [4]"=cluster{u32, u32}[] [{16711680, 16711680}] ("颜色[4]")) -> ()  [unwired: 1 in, 2 out]
                  }
                  frame True {
                    n355 = global read "A131258.vi" "LED-力特性"() -> (w208:refnum<vi>)
                    n356 = property class="Bool"(reference=w208, "Colors [4]"=cluster{u32, u32}[] [{6618880, 6618880}] ("颜色[4]")) -> ()  [unwired: 1 in, 2 out]
                  }
                }
              }
              frame #3 {
                n357 = global read "Global.vi" "试验项目"() -> (w210:bool[])
                n358 = for {
                  tunnel: w210 -> [w211] mode=indexing
                  i -> [w212]
                  n359 = case shown="1" w212 {
                    tunnel: w211 -> [_ w213]
                    frame Default {
                    }
                    frame 1 {
                      n360 = case shown="真" w213 {
                        frame False {
                          n361 = local write "STEP"("内泄露判定" ("STEP")) -> ()
                          n362 = global write "A131258.vi" "试验项"(enum32{"力特性", "内泄露", "压销位移力曲线"}."内泄露" ("试验项")) -> ()
                        }
                        frame True {
                          n363 = local write "STEP"("灵敏度判定" ("STEP")) -> ()
                        }
                      }
                    }
                  }
                }
              }
            }
          }
          frame "灵敏度判定" {
            n364 = stacked-sequence {
              frame #0 {
                n365 = global read "Global.vi" "Result"() -> (w217:refnum<vi>)
                n366 = property class="Tbl"(reference=w217) -> (reference out=w220:refnum<vi>, error out=w227:errorcluster, "Row Headers[]"=w218:string[])  [unwired: 1 in]
                n367 = Build Array (concatenate)(w218, string[] ["灵敏度"] ("数组")) -> (w219:string[])
                n368 = property class="Tbl"(reference=w220, error in=w227, "Row Headers[]"=w219) -> (reference out=w221:refnum<vi>, error out=w228:errorcluster)
                n369 = property class="Tbl"(reference=w221, error in=w228) -> (reference out=w223:refnum<vi>, error out=w229:errorcluster, "Value"=w224:string[][])
                n370 = Build Array (concatenate)(w224, string[][] [[" "]] ("数组")) -> (w225:string[][])
                n371 = property class="Tbl"(reference=w223, error in=w229, "Value"=w225) -> ()  [unwired: 2 out]
              }
              frame #1 {
                n372 = global read "A131258.vi" "灵敏度曲线"() -> (w232:refnum<vi>)
                n373 = global read "A131258.vi" "灵敏度"() -> (w231:T4)
                n374 = call "灵敏度判定.vi"("曲线引用"=w232, "灵敏度"=w231) -> ("OK？"=w230:bool)  [unwired: 6 in, 2 out]
                n375 = case shown="假" w230 {
                  frame False {
                    n376 = local write "合格"(FALSE ("合格")) -> ()
                    n377 = global read "A131258.vi" "LED-灵敏度"() -> (w234:refnum<vi>)
                    n378 = property class="Bool"(reference=w234, "Colors [4]"=cluster{u32, u32}[] [{16711680, 16711680}] ("颜色[4]")) -> ()  [unwired: 1 in, 2 out]
                  }
                  frame True {
                    n379 = global read "A131258.vi" "LED-灵敏度"() -> (w236:refnum<vi>)
                    n380 = property class="Bool"(reference=w236, "Colors [4]"=cluster{u32, u32}[] [{6618880, 6618880}] ("颜色[4]")) -> ()  [unwired: 1 in, 2 out]
                  }
                }
              }
              frame #2 {
                n381 = local write "STEP"("内泄露判定" ("STEP")) -> ()
                n382 = global write "A131258.vi" "试验项"(enum32{"力特性", "内泄露", "压销位移力曲线"}."内泄露" ("试验项")) -> ()
              }
            }
          }
          frame "内泄露判定" {
            n383 = stacked-sequence {
              frame #0 {
                n384 = global read "Global.vi" "Result"() -> (w240:refnum<vi>)
                n385 = property class="Tbl"(reference=w240) -> (reference out=w243:refnum<vi>, error out=w250:errorcluster, "Row Headers[]"=w241:string[])  [unwired: 1 in]
                n386 = Build Array (concatenate)(w241, string[] ["内泄露"] ("数组")) -> (w242:string[])
                n387 = property class="Tbl"(reference=w243, error in=w250, "Row Headers[]"=w242) -> (reference out=w244:refnum<vi>, error out=w251:errorcluster)
                n388 = property class="Tbl"(reference=w244, error in=w251) -> (reference out=w246:refnum<vi>, error out=w252:errorcluster, "Value"=w247:string[][])
                n389 = Build Array (concatenate)(w247, string[][] [[" "]] ("数组")) -> (w248:string[][])
                n390 = property class="Tbl"(reference=w246, error in=w252, "Value"=w248) -> ()  [unwired: 2 out]
              }
              frame #1 {
                n391 = global read "A131258.vi" "内泄露曲线"() -> (w255:refnum<vi>)
                n392 = global read "A131258.vi" "内泄露"() -> (w254:cluster{"下限":dbl, "上限":dbl})
                n393 = call "内泄露.vi"("曲线引用"=w255, "内泄露"=w254) -> ("OK？"=w253:bool)  [unwired: 6 in, 2 out]
                n394 = case shown="假" w253 {
                  frame False {
                    n395 = local write "合格"(FALSE ("合格")) -> ()
                    n396 = global read "A131258.vi" "LED-内泄露"() -> (w257:refnum<vi>)
                    n397 = property class="Bool"(reference=w257, "Colors [4]"=cluster{u32, u32}[] [{16711680, 16711680}] ("颜色[4]")) -> ()  [unwired: 1 in, 2 out]
                  }
                  frame True {
                    n398 = global read "A131258.vi" "LED-内泄露"() -> (w259:refnum<vi>)
                    n399 = property class="Bool"(reference=w259, "Colors [4]"=cluster{u32, u32}[] [{6618880, 6618880}] ("颜色[4]")) -> ()  [unwired: 1 in, 2 out]
                  }
                }
              }
              frame #2 {
                n400 = local write "STEP"("试验项-自由间隙" ("STEP")) -> ()
              }
            }
          }
          frame "自由间隙判定" {
            n401 = stacked-sequence {
              frame #0 {
                n402 = global read "Global.vi" "Result"() -> (w262:refnum<vi>)
                n403 = property class="Tbl"(reference=w262) -> (reference out=w265:refnum<vi>, error out=w272:errorcluster, "Row Headers[]"=w263:string[])  [unwired: 1 in]
                n404 = Build Array (concatenate)(w263, string[] ["自由间隙"] ("数组")) -> (w264:string[])
                n405 = property class="Tbl"(reference=w265, error in=w272, "Row Headers[]"=w264) -> (reference out=w266:refnum<vi>, error out=w273:errorcluster)
                n406 = property class="Tbl"(reference=w266, error in=w273) -> (reference out=w268:refnum<vi>, error out=w274:errorcluster, "Value"=w269:string[][])
                n407 = Build Array (concatenate)(w269, string[][] [[" "]] ("数组")) -> (w270:string[][])
                n408 = property class="Tbl"(reference=w268, error in=w274, "Value"=w270) -> ()  [unwired: 2 out]
              }
              frame #1 {
                n409 = global read "A131258.vi" "自由间隙曲线"() -> (w277:refnum<vi>)
                n410 = global read "A131258.vi" "自由间隙"() -> (w276:cluster{"下限":dbl, "上限":dbl})
                n411 = call "自由间隙.vi"("曲线引用"=w277, "自由间隙判定条件"=w276) -> ("OK？"=w275:bool)  [unwired: 6 in, 2 out]
                n412 = case shown="假" w275 {
                  frame False {
                    n413 = local write "合格"(FALSE ("合格")) -> ()
                    n414 = global read "A131258.vi" "LED-自由间隙"() -> (w279:refnum<vi>)
                    n415 = property class="Bool"(reference=w279, "Colors [4]"=cluster{u32, u32}[] [{16711680, 16711680}] ("颜色[4]")) -> ()  [unwired: 1 in, 2 out]
                  }
                  frame True {
                    n416 = global read "A131258.vi" "LED-自由间隙"() -> (w281:refnum<vi>)
                    n417 = property class="Bool"(reference=w281, "Colors [4]"=cluster{u32, u32}[] [{6618880, 6618880}] ("颜色[4]")) -> ()  [unwired: 1 in, 2 out]
                  }
                }
              }
              frame #2 {
                n418 = shared-variable "我的电脑\\A131258.lvlib\\设备状态"(i16 40 ("设备状态")) -> ()  [unwired: 1 in, 1 out]
                n419 = local write "STEP"("等待" ("STEP")) -> ()
              }
            }
          }
          frame "不合格锁定" {
            n420 = call "临时授权.vi"() -> ("授权成功"=w286:bool)  [unwired: 11 in]
            n421 = Wait (ms)(milliseconds to wait=u32 100 ("等待时间（毫秒）")) -> ()  [unwired: 1 out]
            n422 = case shown="真" w286 {
              frame False {
              }
              frame True {
                n423 = local write "STEP"("报表" ("STEP")) -> ()
                n424 = shared-variable "我的电脑\\A131258.lvlib\\设备状态"(i16 3722 ("设备状态")) -> ()  [unwired: 1 in, 1 out]
              }
            }
          }
          frame "合格判定" {
            n425 = local read "合格"() -> (w290:bool)
            n426 = Wait (ms)(milliseconds to wait=u32 100 ("等待时间（毫秒）")) -> ()  [unwired: 1 out]
            n427 = local write "STEP"("报表" ("STEP")) -> ()
            n428 = call <userlib>:"Boolean Trigger__ogtk.vi"("Boolean Input"=w290) -> ("Rising Edge"=w289:bool)  [unwired: 1 in, 1 out]
            n429 = case shown="真" w289 {
              frame False {
              }
              frame True {
                n430 = global read "Global.vi" "合格数量"() -> (w294:i32)
                n431 = Increment(x=w294) -> (x+1=w293:i32)
                n432 = global write "Global.vi" "合格数量"(w293) -> ()
              }
            }
          }
          frame "报表" {
            n433 = disable-structure shown="启用" {
              frame Disabled {
                n434 = shared-variable "我的电脑\\Global.lvlib\\工位追溯码"() -> (w300:string)  [unwired: 1 in, 1 out]
                n435 = shared-variable "我的电脑\\Global.lvlib\\联机模式"() -> (w301:i16)  [unwired: 1 in, 1 out]
                n436 = call "Report_A131258.vi"("文件重命名"=TRUE, "文件名称"=w300, "布尔数组"="判定结果") -> ("error out"=w297:errorcluster)  [unwired: 8 in]
                n437 = case shown="1" w301 {
                  tunnel: w297 -> [_ w302]
                  frame 0, Default {
                  }
                  frame 1 {
                    n438 = call "上传数据库.vi"("错误输入"=w302) -> ()  [unwired: 10 in, 1 out]
                  }
                }
              }
              frame Enabled {
                n439 = call "走合数据.vi"("Type"=enum16{"Write", "Read"}."Read") -> ("error out"=w303:errorcluster)  [unwired: 9 in, 1 out]
                n440 = call "Report.vi"("error in (no error)"=w303) -> ()  [unwired: 10 in, 1 out]
              }
            }
            n441 = shared-variable "我的电脑\\A131258.lvlib\\设备状态"() -> (w295:i16)  [unwired: 1 in, 1 out]
            n442 = call "浮动通知.vi"("通知内容"="报表生成中" ("Status")) -> ()  [unwired: 11 in]
            n443 = case shown="默认" w295 {
              frame Default {
                n444 = local write "STEP"("等待启动" ("STEP")) -> ()
              }
              frame 3721..3723 {
                n445 = local write "STEP"("等待" ("STEP")) -> ()
              }
            }
          }
        }
        n446 = global read "Global.vi" "程序关闭"() -> (w15:bool)
      }
    }
  }
